vi "CurrentSetY.vi"(10 "Cluster":T1={"VISA resource name"="COM6", "baud rate (9600)"=9600, "data bits (8)"=8, "parity (0:none)"=enum."None"} {"data bits (8)" min=5 max=8 step=1}, 11 "电流设置":dbl min=-5.0 max=5.0 step=0.2) -> ()   [LabVIEW 2020, in "YP03-60CurrentSource_1.lvlib"]
uses:
  YP03-60CurrentSource_1.lvlib
  <vilib>/Instr/_visa.llb/VISA Configure Serial Port (Instr).vi
panel:
  in  "error in (no error)":errorcluster
  out "error out":errorcluster
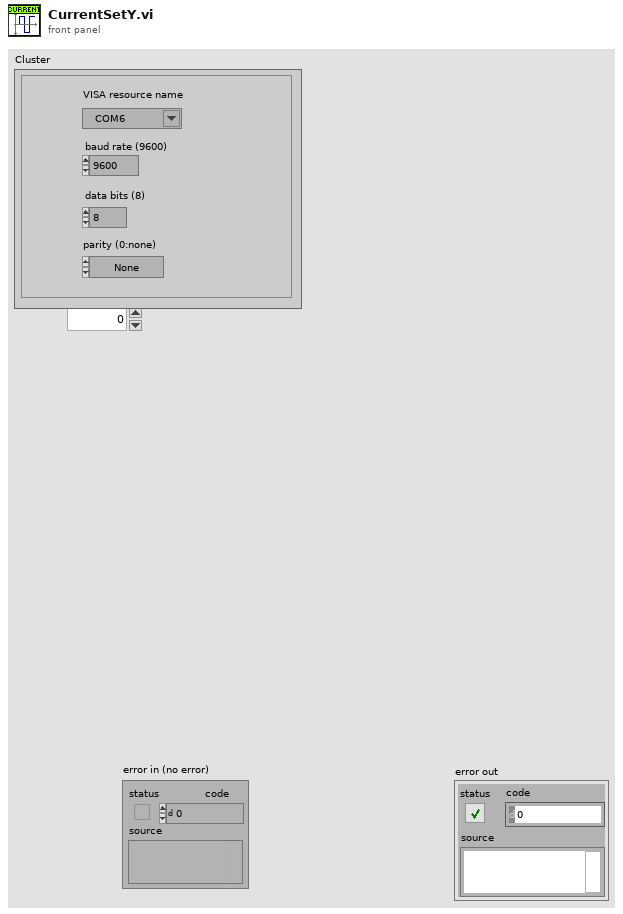
[diagram p1: front panel]
types:
  T1 = cluster{"VISA resource name":refnum<visa-resource-name>, "baud rate (9600)":u32, "data bits (8)":u16, "parity (0:none)":enum16{"None", "Odd", "Even", "Mark", "Space"}}
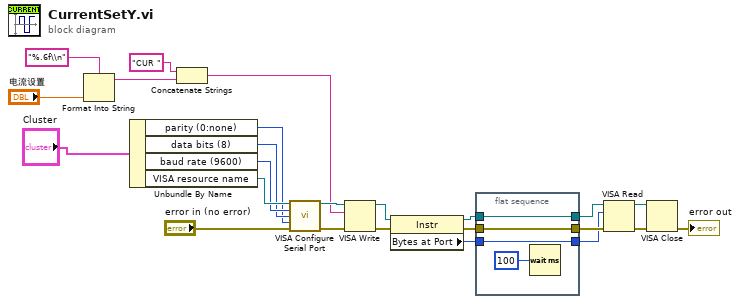
[diagram p0: block diagram]
diagram:
  n1 = Format Into String(format string="%.6f\\n", "电流设置") -> (resulting string=w9:string)  [unwired: 2 in, 1 out]
  n2 = Unbundle By Name("Cluster") -> ("parity (0:none)"=w2:enum16{"None", "Odd", "Even", "Mark", "Space"}, "data bits (8)"=w3:u16, "baud rate (9600)"=w4:u32, "VISA resource name"=w5:refnum<visa-resource-name>)
  n3 = Concatenate Strings("CUR " ("string"), w9) -> (w13:string)
  n4 = call-poly "VISA Configure Serial Port"("VISA resource name"=w5, "baud rate (9600)"=w4, "data bits (8)"=w3, "parity (0:none)"=w2, "error in (no error)"="error in (no error)") -> ("VISA resource name out"=w20:refnum<visa-resource-name>, "error out"=w21:errorcluster)  [unwired: 9 in]
  n5 = VISA Write(VISA resource name=w20, write buffer=w13, error in (no error)=w21) -> (VISA resource name out=w11:refnum<visa-resource-name>, error out=w12:errorcluster)  [unwired: 1 out]
  n6 = property class="Instr"(reference=w11, error in=w12) -> (reference out=w16:refnum<visa-resource-name>, error out=w18:errorcluster, "Bytes at Port"=w14:u32)
  n7 = flat-sequence {
    tunnel: w16 -> [w28]
    tunnel: [w28] -> w17
    tunnel: [w27] -> w19
    tunnel: w18 -> [w27]
    tunnel: [w26] -> w15
    tunnel: w14 -> [w26]
    frame #0 {
      n8 = Wait (ms)(milliseconds to wait=u32 100) -> ()  [unwired: 1 out]
    }
  }
  n9 = VISA Read(VISA resource name=w17, byte count=w15, error in (no error)=w19) -> (VISA resource name out=w24:refnum<visa-resource-name>, error out=w23:errorcluster)  [unwired: 2 out]
  n10 = VISA Close(VISA resource name=w24, error in (no error)=w23) -> (error out=→"error out":errorcluster)
